vi "ILD_15 graph.vi"(8 "标题.文本":string, 9 "Limit Data":cluster{"Frequency":dbl[], "Data In":dbl[]}[](array[cluster]), 10 "Graph Index":i32, 11 "Test Graph":refnum<vi>[](array[refnum])=[refnum, refnum, refnum, refnum, refnum, refnum, refnum, refnum, refnum, refnum]) -> ()   [LabVIEW 2011]
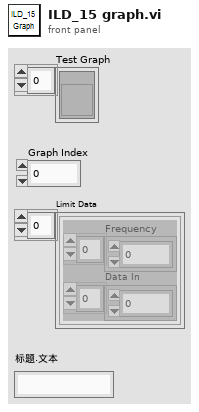
[diagram p1: front panel]
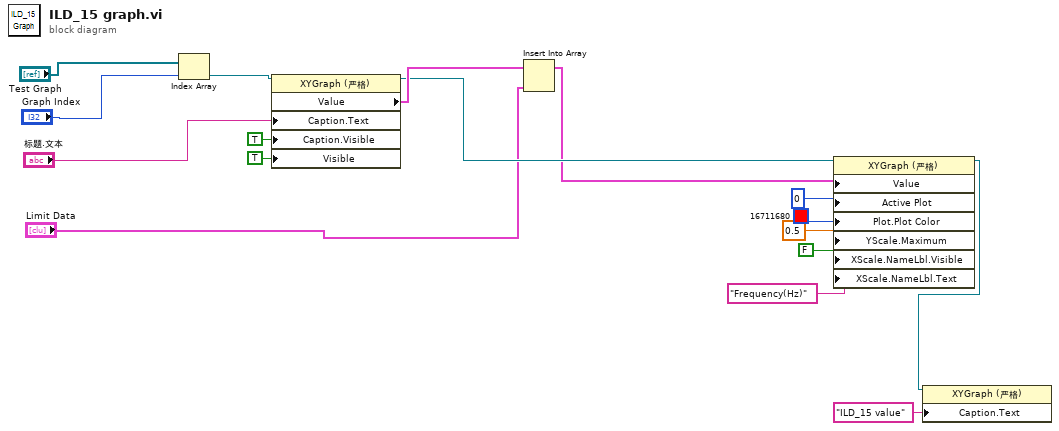
[diagram p0: block diagram]
diagram:
  n1 = Index Array(array="Test Graph", index="Graph Index") -> (element=w15:refnum<vi>)
  n2 = property class="XYGraph (严格)"(reference=w15, "Caption.Text"="标题.文本", "Caption.Visible"=TRUE ("标题.可见"), "Visible"=TRUE ("可见")) -> (reference out=w10:refnum<vi>, "Value"=w11:cluster{"Horz Time array":dbl[], "Y":dbl[]}[])  [unwired: 1 in, 1 out]
  n3 = Insert Into Array(array=w11, new element="Limit Data") -> (w9:cluster{"Horz Time array":dbl[], "Y":dbl[]}[])  [unwired: 1 in]
  n4 = property class="XYGraph (严格)"(reference=w10, "Value"=w9, "Active Plot"=u32 0 ("活动曲线"), "Plot.Plot Color"=u32 16711680, "YScale.Maximum"=0.5 ("Y标尺.范围:最大值"), "XScale.NameLbl.Visible"=FALSE ("X标尺.名称标签.可见"), "XScale.NameLbl.Text"="Frequency(Hz)" ("X标尺.名称标签.文本")) -> (reference out=w3:refnum<vi>)  [unwired: 1 in, 1 out]
  n5 = property class="XYGraph (严格)"(reference=w3, "Caption.Text"="ILD_15 value" ("标题.文本")) -> ()  [unwired: 1 in, 2 out]
